vi "Motor Command with Limit Switches.vi"(1 "LowLimitSwitch":bool, 2 "MotorCommandIn":dbl(slide) scale=-1.0..1.0, 3 "HighLimitSwitch":bool) -> (0 "?":dbl)   [LabVIEW 2017]
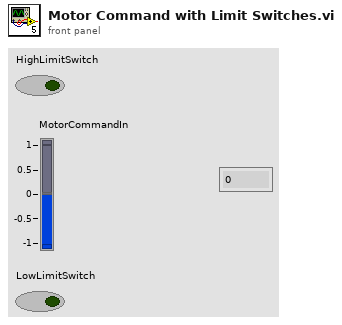
[diagram p1: front panel]
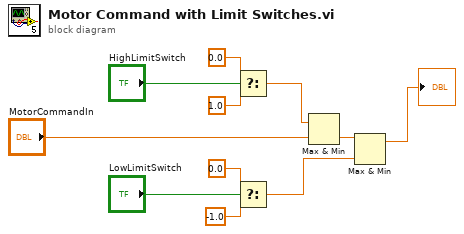
[diagram p0: block diagram]
diagram:
  n1 = Select(t=0.0, s="HighLimitSwitch", f=1.0) -> (s? t:f=w5:dbl)
  n2 = Select(t=0.0, s="LowLimitSwitch", f=-1.0) -> (s? t:f=w3:dbl)
  n3 = Max & Min(x=w5, y="MotorCommandIn") -> (min(x,y)=w2:dbl)  [unwired: 1 out]
  n4 = Max & Min(x=w2, y=w3) -> (max(x,y)=→"?":dbl)  [unwired: 1 out]
